vi "Dashboard Main.vi"() -> ()   [LabVIEW 2015]
uses:
  <vilib>/Utility/miscctls.llb/LVRowAndColumnTypeDef.ctl
  <vilib>/event_ctls.llb/eventvkey.ctl
  <vilib>/Rock Robotics/WPI/Dashboard/WPI_DashboardLogging Global.vi
  <vilib>/Rock Robotics/Network Tables/NT Read Numeric Array.vi
  <vilib>/Utility/config.llb/Write Key (String).vi
  <vilib>/Utility/config.llb/Write Key (I32).vi
  <vilib>/Utility/config.llb/NI_LVConfig.lvlib
panel:
  in  "TCP":refnum<k5>
  in  "Rec Mode":enum32{"Stop", "Record", "Playback"}(radio)
  in  "Vision":u16(ring) items=["Camera Off", "USB Camera SW", "USB Camera HW", "IP Camera"]
  out "Camera IP":string
  out "Image Message":string="Timeout in Camera Communications"
  in  "Dashboard Tab":T1(tab)
  in  "Select Auto":string(combo)
  out "NT Connection":bool
  in  "Camera Settings":T2={"Frame Rate"=30, "Compression"=30, "Size"=1} {"Frame Rate" scale=1.0..30.0; "Size" items=["640x480", "320x240", "160x120"]}
  out "MotorChart R":cluster{"Numeric":dbl, "Numeric":dbl}(graph)
  out "MotorChart L":T3(graph)
  out "MotorSliders R":cluster{"MotorSlide1":dbl, "MotorSlide2":dbl} {"MotorSlide2" scale=-1.0..1.0 scale format="%#_2e"; "MotorSlide1" scale=-1.0..1.0 scale format="%#_2e"}
  out "MotorSliders L":T4 {"MotorSlide4 2" scale=0.0..14.0 scale format="%#_2e"; "MotorSlide2" scale=-1.0..1.0 scale format="%#_2e"; "MotorSlide1" scale=-1.0..1.0 scale format="%#_2e"}
  out "Gyro":dbl(knob) scale=0.0..360.0
  out "JS1 Z":dbl(slide) scale=-1.0..1.0 scale format="%#_2e"
  out "JS1 Graph":cluster{"X":dbl, "Y":dbl}[](graph)
  out "JS1 Buttons":T5
  out "JS2 Z":dbl(slide) scale=-1.0..1.0 scale format="%#_2e"
  out "JS2 Graph":cluster{"X":dbl, "Y":dbl}[](graph)
  out "JS2 Buttons":T5
  out "Mode":T6(ring)=enum."Auto Disabled"
  in  "DB Camera Config":bool
  out "fps":dbl format="%#.1g"
  out "Mbps":dbl format="%#.1g"
  out "Mbps LED":bool
  in  "DB/String 9":string
  in  "DB/String 8":string
  in  "DB/String 7":string
  in  "DB/String 6":string
  in  "DB/String 5":string
  in  "DB/String 4":string
  in  "DB/String 3":string
  in  "DB/String 2":string
  in  "DB/String 1":string
  in  "DB/String 0":string
  in  "DB/Slider 0":dbl(slide) scale=0.0..5.0
  in  "DB/Slider 1":dbl(slide) scale=0.0..5.0
  in  "DB/Slider 2":dbl(slide) scale=0.0..5.0
  in  "DB/Slider 3":dbl(slide) scale=0.0..5.0
  out "DB/LED 3":bool
  out "DB/LED 2":bool
  out "DB/LED 1":bool
  out "DB/LED 0":bool
  in  "DB/Button 3":bool
  in  "DB/Button 2":bool
  in  "DB/Button 1":bool
  in  "DB/Button 0":bool caption="New Name"
  in  "Position_y":dbl
  in  "Position_x":dbl
  out "XY Graph":cluster{"X":dbl[], "Y":dbl[]}[](graph)
  in  "Reset_Camera":bool=TRUE
  in  "Enable_Camera":bool=TRUE
  in  "Test Slider":dbl(slide) scale=0.0..100.0 scale format="%#_3g"
  in  "On/Off":bool caption="Solenoid"
  in  "Test Name":u16(ring) items=["Select the test to run..."]
  in  "Test Tree":string(tree)
  in  "Motor":cluster{"Value":dbl, "Enable":bool} {"Value" scale=-1.0..1.0 scale format="%#_3g"}
  out "Progress":T7 {"Test Progress" scale=0.0..100.0}
  in  "Rev/Fwd":cluster{"Forward":bool, "Reverse":bool}
  in  "Test Ring":u16(ring) items=["Monochrome", "Color"]
  out "Cmd Status":string
  in  "Execute Command":bool
  in  "Command Params":string[][](table)
  in  "Command Selection":i32(listbox)
  in  "CheckList":i32(listbox)
  out "Tree":string(tree)
  out "Camera Image":T8(plugin-control)
  out "Background":bool
  # "Left"
  # "Front"
  # "Right"
  # "Battery"
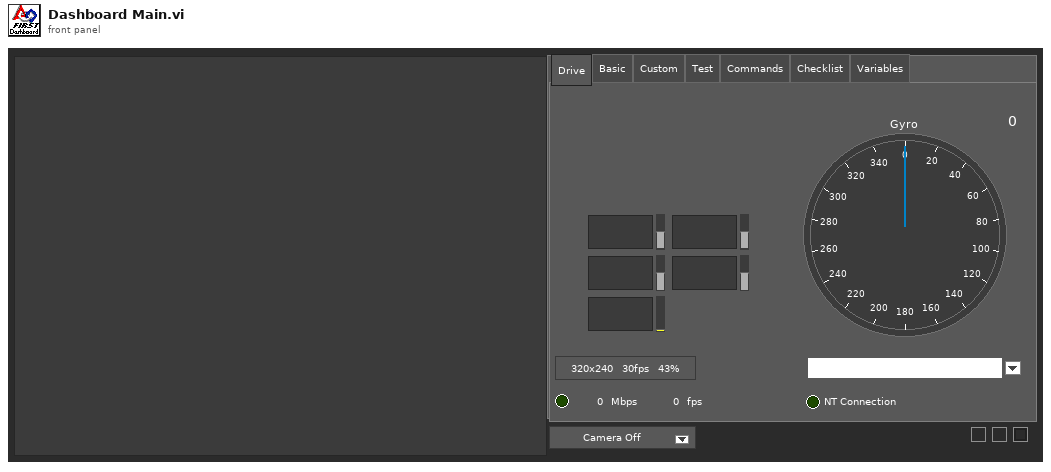
[diagram p1: front panel]
types:
  T1 = enum32{"Drive", "Basic", "Custom", "Test", "Commands", "Checklist", "Variables"}
  T2 = cluster{"Frame Rate":i32, "Compression":i32, "Size":u16}
  T3 = cluster{"Numeric":dbl, "Numeric":dbl, "Battery V":dbl}
  T4 = cluster{"MotorSlide1":dbl, "MotorSlide2":dbl, "MotorSlide4 2":dbl}
  T5 = cluster{bool, bool, bool, bool, bool, bool, bool, bool, bool, bool, bool, bool}
  T6 = enum8{"Tele-Op Disabled", "Tele-Op Enabled", "Auto Disabled", "Auto Enabled", "Test Disabled", "Test Enabled", "Disconnected", "No Code", "E-Stop"}
  T7 = cluster{"Test Progress":u8, "Test Progress Text":string}
  T8 = typedef "IMAQ Image.ctl" = refnum<image>
  T9 = cluster{"IDs":cluster{"RPC field ID":u16, "Unique ID":u16}, "String":string}
  T10 = enum32{"Drive", "Basic", "Custom", "Test", "Checklist", "Variables"}
  T11 = typedef "Image Type" = u32
  T12 = cluster{"Camera Image":refnum<vi>, "Dashboard Tab":refnum<vi>, "Background":refnum<vi>, "Vision":refnum<vi>, "Rec Mode":refnum<vi>, "Test Slider":refnum<vi>, "On/Off ":refnum<vi>, "Test Ring":refnum<vi>, "Rev/Fwd":refnum<vi>, "Test Name":refnum<vi>, "Motor":refnum<vi>, "Progress":refnum<vi>, "CheckList":refnum<vi>, "Tree":refnum<vi>, "Test Tree":refnum<vi>, "Command Params":refnum<vi>, "Command Selection":refnum<vi>, "Execute Command":refnum<vi>, "Cmd Status":refnum<vi>}
  T13 = cluster{"Error Strings":string, "Disable Counts":cluster{u16, u16}, "Rail Faults":cluster{u16, u16, u16}, "Robot IP":string, "DB Mode":u8, "Event Info":cluster{"Name":string, "Type":u8, "Number":u16, "Replay":u8}, "Camera Addr":string}
  T14 = cluster{"Storage":cluster{"Disk Free":u64, "RAM Block":u32, "RAM free":u32}, "CPU Utilization":cluster{"CPU % ISR":sgl, "CPU % Time Crit":sgl, "CPU % Timed Str":sgl, "CPU % High":sgl, "CPU % Above":sgl, "CPU % Normal":sgl, "CPU % Low":sgl}, "CAN":cluster{"% Bus Utilization":sgl, "Bus Off Cnt":u32, "TX_FIFO Full Cnt":u32, "Receive Error Cnt":u8, "Transmit Error Cnt":u8}, "HID":cluster{"HID Outputs":u32, "Rumble Low":u16, "Rumble High":u16}[]}
  T15 = cluster{"Status bits":cluster{"Test Mode":bool, "Autonomous":bool, "Enabled":bool, "Code Start":bool, "Brownout":bool, "Reserved 2":bool, "Reserved 3":bool, "E-Stop":bool}, "Code Trace":cluster{"Disabled":bool, "TeleOp":bool, "Auto":bool, "Test":bool}, "Controller Type":enum16{"unknown", "cRIO", "roboRio"}, "Code?":enum16{"unknown", "noCode", "code"}, "Battery V":dbl}
  T16 = cluster{"Control Bits":cluster{"TestMode":bool, "Autonomous":bool, "Enabled":bool, "FMS Present":bool, bool, bool, bool, "E-Stop":bool}, "Team Station ":u8, "Countdown":sgl, "Joystick Values":cluster{"Axes":dbl[], "Buttons":bool[], "POVs":i16[]}[]}
  T17 = cluster{"Axes":dbl[], "Buttons":bool[], "POVs":i16[]}[]
  T18 = cluster{"Axes":dbl[], "Buttons":bool[], "POVs":i16[]}
  T19 = cluster{"Buttons[0]":bool, "Buttons[1]":bool, "Buttons[2]":bool, "Buttons[3]":bool, "Buttons[4]":bool, "Buttons[5]":bool, "Buttons[6]":bool, "Buttons[7]":bool, "Buttons[8]":bool, "Buttons[9]":bool, "Buttons[10]":bool, "Buttons[11]":bool}
  T20 = typedef "NI_LVConfig.lvlib/Config Data RefNum.ctl" = refnum<k1>
  T21 = cluster{"Operation":enum16{"Update", "Clear"}, "Color Box":u32}[]
  T22 = typedef "eventvkey.ctl" = enum16{"ASCII", "Enter", "Return", "Shift", "Ctrl", "Alt", "Cmd", "Opt", "Caps", "NumLock", "Clear", "Break", "Up", "Down", "Left", "Right", "Insert", "Delete", "Home", "End", "PageUp", "PageDown", "Escape", "Help", "Pause", "ScrollLock", "F1", "F2", "F3", "F4", "F5", "F6", "F7", "F8", "F9", "F10", "F11", "F12", "F13", "F14", "F15", "F16", "F17", "F18", "F19", "F20", "F21", "F22", "F23", "F24", "Play", "VolumeUp", "VolumeDown", "Mute", "Two Byte Char"}
  T23 = cluster{"Image Size":bool, "Image Type":bool, "Pixel Value":bool, "ROI Information":bool, "Zoom Factor":bool}
  T24 = enum8{"Enabled", "Disabled", "Disabled and Grayed Out"}
  T25 = cluster{"Operation":enum16{"Update", "Clear"}, "Color Box":u32}
  T26 = typedef "LVRowAndColumnTypeDef.ctl" = cluster{"Row":i32, "Column":i32}
  T27 = cluster{"Shift":bool, "Ctrl":bool, "Alt":bool, "Cmd":bool, "Opt":bool}
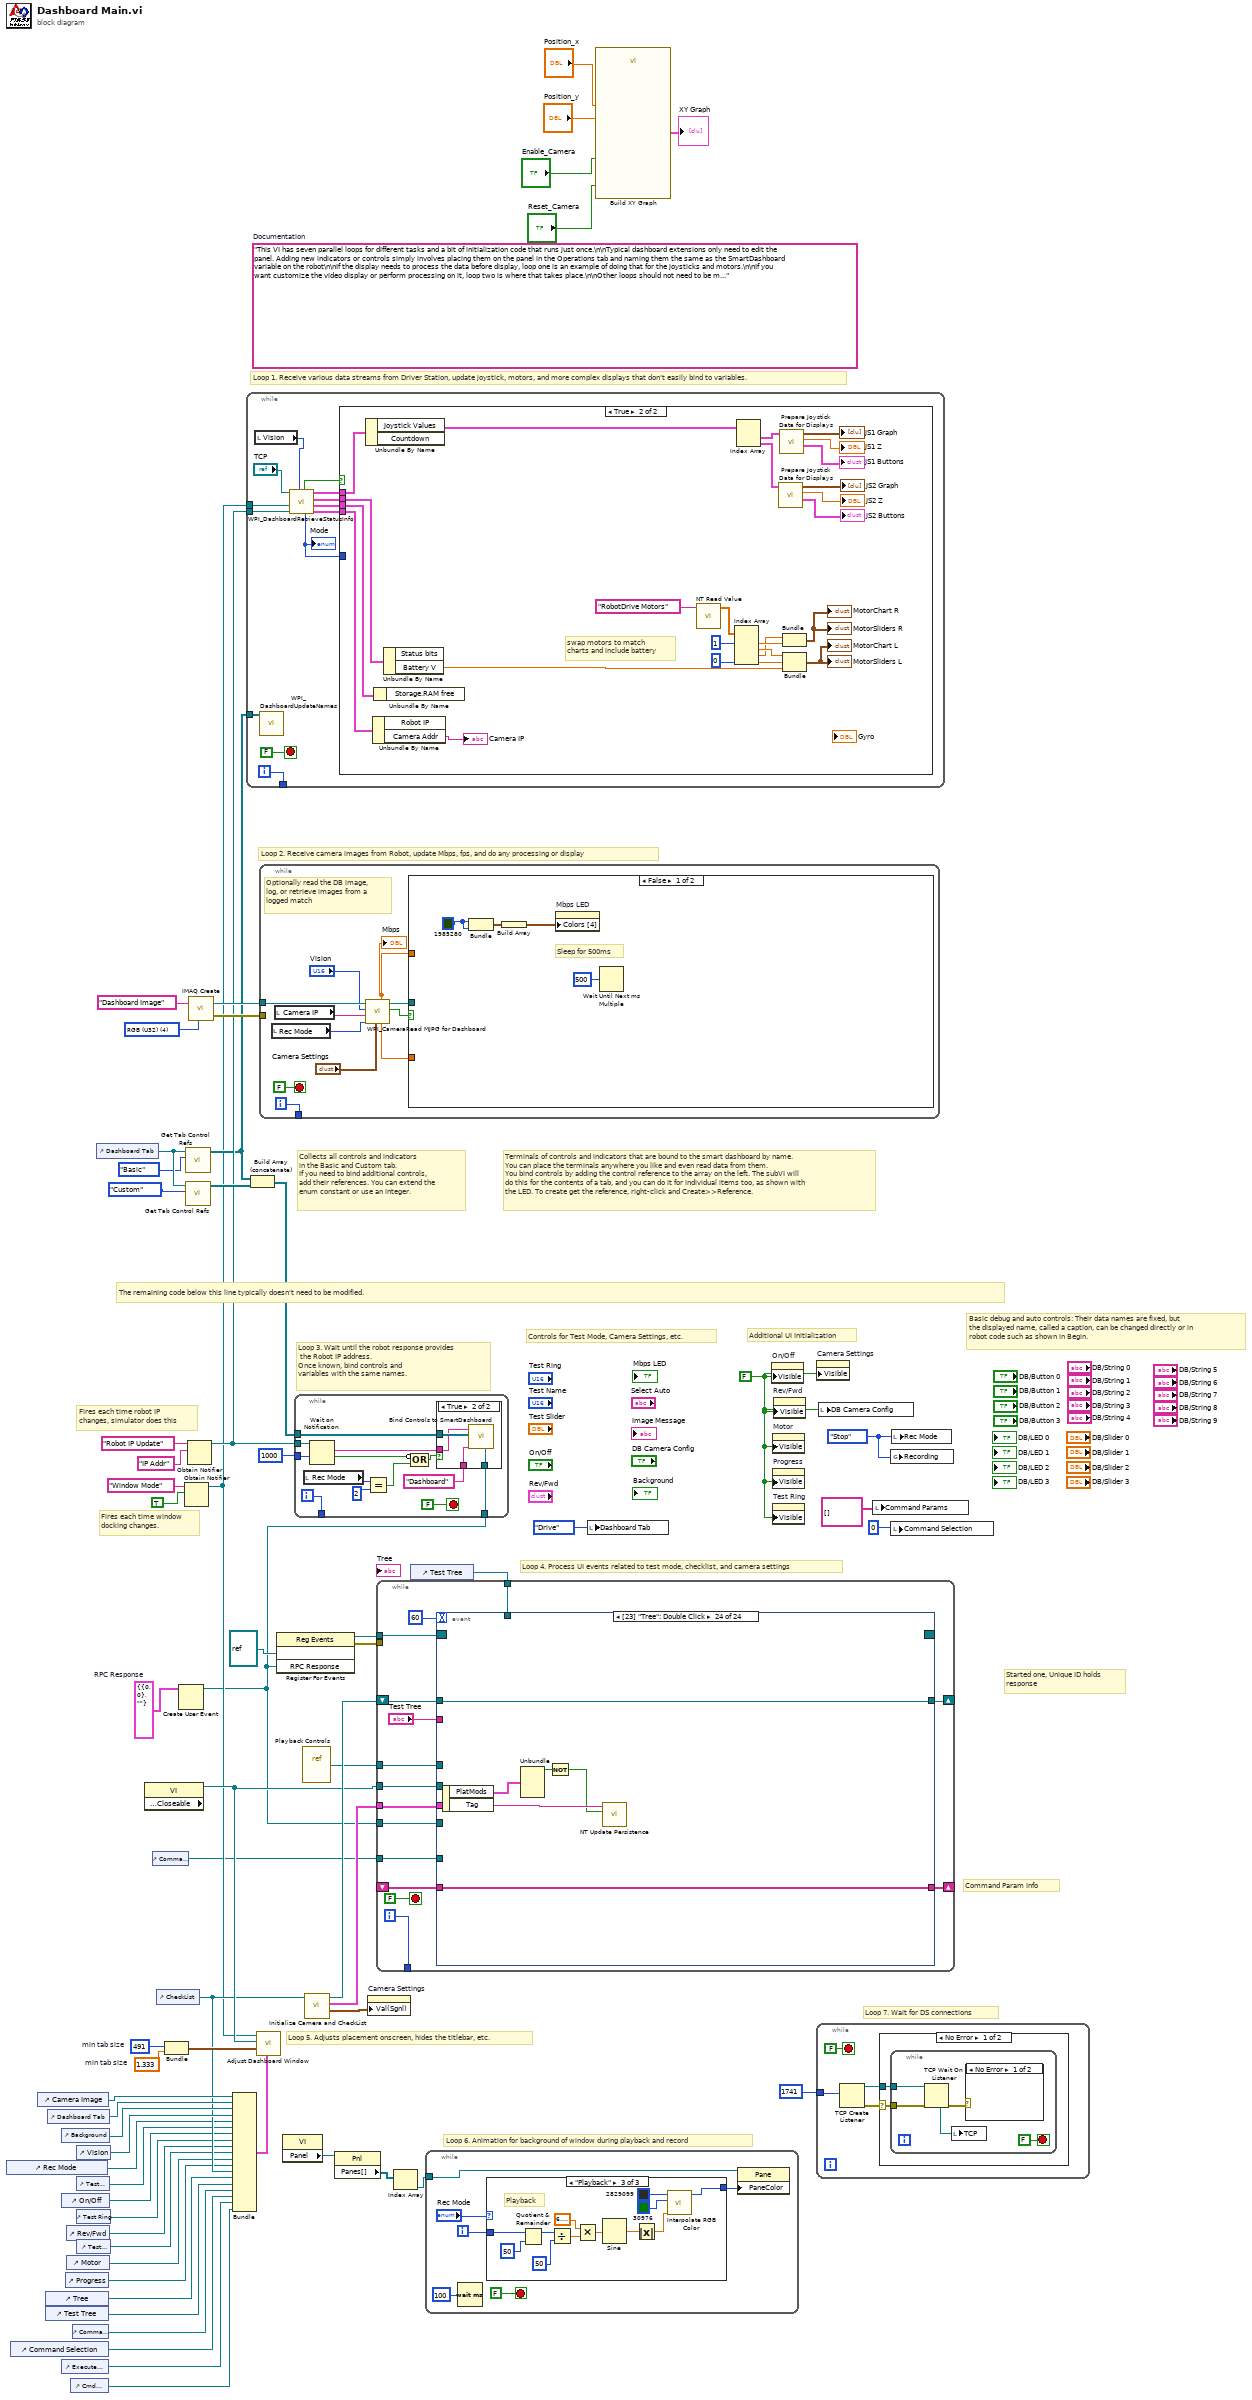
[diagram p0: block diagram]
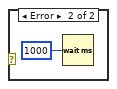
[diagram p2: hidden frame]
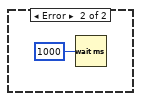
[diagram p3: hidden frame]
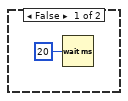
[diagram p4: hidden frame]
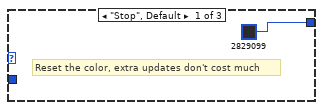
[diagram p5: hidden frame]
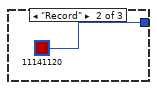
[diagram p6: hidden frame]
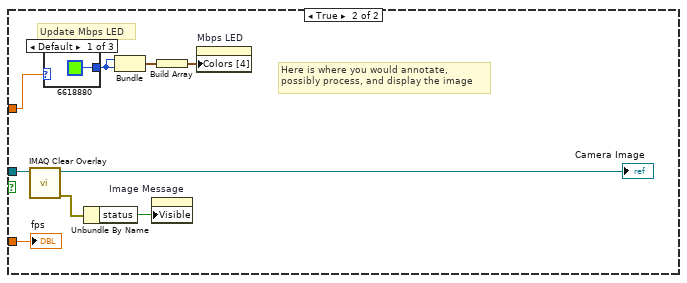
[diagram p8: hidden frame]
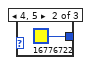
[diagram p9: hidden frame]
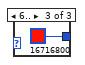
[diagram p10: hidden frame]
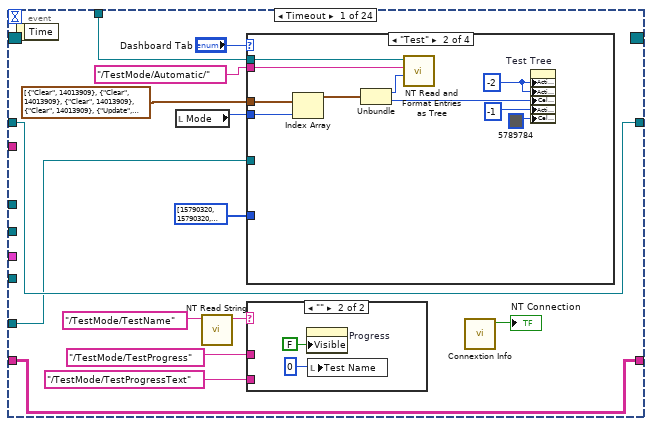
[diagram p11: hidden frame]
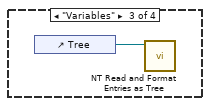
[diagram p13: hidden frame]
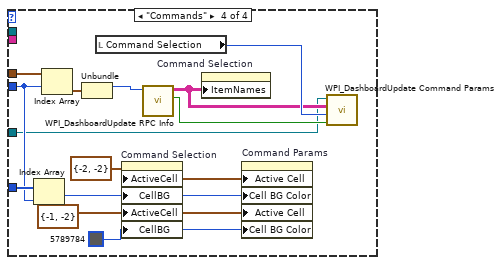
[diagram p14: hidden frame]
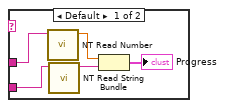
[diagram p15: hidden frame]
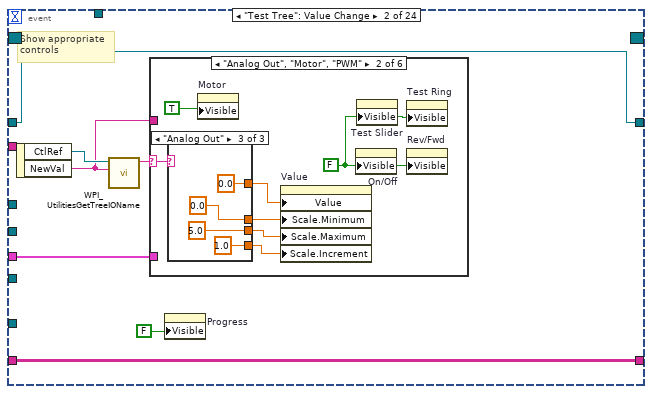
[diagram p16: hidden frame]
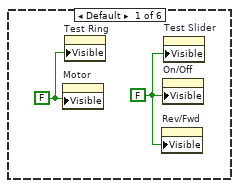
[diagram p17: hidden frame]
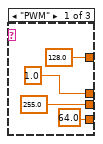
[diagram p18: hidden frame]
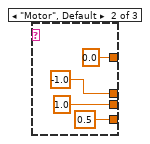
[diagram p19: hidden frame]
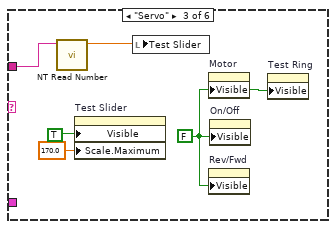
[diagram p20: hidden frame]
diagram:
  w12 = T9 {"IDs"={"RPC field ID"=0, "Unique ID"=0}, "String"=""}  # RPC Response
  w38 = 491  # min tab size
  w37 = 1.333  # min tab size
  w46 = enum32{"Stop", "Record", "Playback"}."Stop" ("Rec Mode")
  w20 = FALSE ("Visible")
  (unwired) "This VI has seven parallel loops for different tasks and a bit of initialization code that runs just once.\n\nTypical dashboard extensions only need to edit the panel. Adding new indicators or controls simply involves placing them on the panel in the Operations tab and naming them the same as the SmartDashboard variable on the robot\n\nIf the display needs to process the data before display, loop one is an example of doing that for the joysticks and motors.\n\nIf you want customize the video display or perform processing on it, loop two is where that takes place.\n\nOther loops should not need to be modified. They are pretty standard, and document the task they perform."  # Documentation
  w66 = T11 4 items=["Grayscale (U8)", "Grayscale (I16)", "Grayscale (SGL)", "Complex (CSG)", "RGB (U32)", "HSL (U32)", "RGB (U64)"] ("Image Type")
  # "Command Param Info"
  # "Started one, Unique ID holds\nresponse"
  # "Loop 7. Wait for DS connections"
  # "Basic debug and auto controls: Their data names are fixed, but\nthe displayed name, called a caption, can be changed directly or in\nrobot code such as shown in Begin."
  # "Controls for Test Mode, Camera Settings, etc."
  # "Additional UI Initialization"
  # "Loop 6. Animation for background of window during playback and record"
  # "Fires each time robot IP\nchanges, simulator does this"
  # "Fires each time window\ndocking changes."
  # "Collects all controls and indicators\nin the Basic and Custom tab.\nIf you need to bind additional controls,\nadd their references. You can extend the\nenum constant or use an integer."
  # "The remaining code below this line typically doesn't need to be modified."
  # "Loop 4. Process UI events related to test mode, checklist, and camera settings"
  # "Terminals of controls and indicators that are bound to the smart dashboard by name.\nYou can place the terminals anywhere you like and even read data from them.\nYou bind controls by adding the control reference to the array on the left. The subVI will\ndo this for the contents of a tab, and you can do it for individual items too, as shown with\nthe LED. To create get the reference, right-click and Create>>Reference."
  # "Loop 3. Wait until the robot response provides\n the Robot IP address.\nOnce known, bind controls and\nvariables with the same names."
  # "Loop 5. Adjusts placement onscreen, hides the titlebar, etc."
  # "Loop 1. Receive various data streams from Driver Station, update joystick, motors, and more complex displays that don't easily bind to variables."
  # "Loop 2. Receive camera images from Robot, update Mbps, fps, and do any processing or display"
  n1 = control-ref of="Rec Mode"() -> (w26:refnum<vi>)
  n2 = control-ref of="Command Selection"() -> (w11:refnum<vi>)
  n3 = control-ref of="Camera Image"() -> (w41:refnum<vi>)
  n4 = control-ref of="Tree"() -> (w30:refnum<vi>)
  n5 = control-ref of="Test Tree"() -> (w29:refnum<vi>)
  n6 = control-ref of="Dashboard Tab"() -> (w40:refnum<vi>)
  n7 = control-ref of="Execute Command"() -> (w13:refnum<vi>)
  n8 = control-ref of="Background"() -> (w35:refnum<vi>)
  n9 = control-ref of="On/Off"() -> (w24:refnum<vi>)
  n10 = control-ref of="Progress"() -> (w21:refnum<vi>)
  n11 = control-ref of="Rev/Fwd"() -> (w22:refnum<vi>)
  n12 = control-ref of="Motor"() -> (w27:refnum<vi>)
  n13 = control-ref of="Cmd Status"() -> (w7:refnum<vi>)
  n14 = control-ref of="Command Params"() -> (w14:refnum<vi>)
  n15 = control-ref of="Test Slider"() -> (w25:refnum<vi>)
  n16 = control-ref of="Vision"() -> (w39:refnum<vi>)
  n17 = control-ref of="Test Ring"() -> (w23:refnum<vi>)
  n18 = control-ref of="Test Name"() -> (w28:refnum<vi>)
  n19 = control-ref of="Dashboard Tab"() -> (w44:refnum<vi>)
  n20 = property class="VI" props=["Front Panel.Closeable"]() -> (reference out=w45:refnum<vi>)  [unwired: 2 in, 2 out]
  n21 = control-ref of="Command Params"() -> (w6:refnum<vi>)
  n22 = control-ref of="CheckList"() -> (w31:refnum<vi>)
  n23 = Bundle("min tab size"=w38, "min tab size"=w37) -> (w36:cluster{"min tab size":i32, "min tab size":dbl})  [unwired: 1 in]
  n24 = Create User Event(user event datatype=w12) -> (user event=w8:refnum<user-event>)  [unwired: 1 in, 1 out]
  n25 = Obtain Notifier(name (unnamed)="Window Mode", notification data type=TRUE) -> (notifier out=w17:refnum<notifier>)  [unwired: 2 in, 2 out]
  n26 = call <vilib>:"Get Tab Control Refs.vi"("Page Index"=T10."Basic" ("Dashboard Tab"), "TabControl in"=w44) -> ("ControlsOnPage"=w18:refnum<vi>[])  [unwired: 9 in]
  n27 = call <vilib>:"Get Tab Control Refs.vi"("Page Index"=T10."Custom" ("Dashboard Tab"), "TabControl in"=w44) -> ("ControlsOnPage"=w43:refnum<vi>[])  [unwired: 9 in]
  n28 = Obtain Notifier(name (unnamed)="Robot IP Update", notification data type="IP Addr" ("name (unnamed)")) -> (notifier out=w19:refnum<notifier>)  [unwired: 2 in, 2 out]
  n29 = call "IMAQ Create"("Image Name"="Dashboard Image", "Image Type"=w66) -> ("New Image"=w64:T8, "error out"=w63:errorcluster)  [unwired: 2 in, 1 out]
  n30 = Bundle("Camera Image"=w41, "Dashboard Tab"=w40, "Background"=w35, "Vision"=w39, "Rec Mode"=w26, "Test Slider"=w25, "On/Off"=w24, "Test Ring"=w23, "Rev/Fwd"=w22, "Test Name"=w28, "Motor"=w27, "Progress"=w21, "CheckList"=w31, "Tree"=w30, "Test Tree"=w29, "Command Params"=w14, "Command Selection"=w11, "Execute Command"=w13, "Cmd Status"=w7) -> (w32:T12)  [unwired: 1 in]
  n31 = while {
    tunnel: [w78] -> _
    tunnel: w19 -> [w72]
    tunnel: w18 -> [w71]
    tunnel: w17 -> [w67]
    i -> [w78]
    stop <- FALSE stop-if-true
    n32 = local read "Vision"() -> (w69:u16)
    n33 = call <vilib>:"WPI_DashboardUpdateNames.vi"("Controls on Tab"=w71) -> ()  [unwired: 11 in]
    n34 = call <vilib>:"WPI_DashboardRetrieveStatusInfo.vi"("Vision"=w69, "Binding Refnum"=w72, "Window Mode Notifier"=w67, "TCP Cnx"="TCP") -> ("Power and Errors"=w73:T13, "Robot Metrics"=w76:T14, "Status Info"=w77:T15, "Control Info"=w74:T16, "Robot Mode"=w70:T6, "Process?"=w75:bool)  [unwired: 2 in]
    "Mode" <- w70
    n35 = case shown="True" w75 {
      tunnel: w77 -> [_ w105]
      tunnel: w76 -> [_ w104]
      tunnel: w74 -> [_ w103]
      tunnel: w73 -> [_ w102]
      tunnel: w70 -> [_ _]
      frame False {
        n36 = Wait (ms)(milliseconds to wait=u32 20) -> ()  [unwired: 1 out]
      }
      frame True {
        # "swap motors to match\ncharts and include battery"
        n37 = Unbundle By Name(w103) -> ("Joystick Values"=w92:T17)  [unwired: 1 out]
        n38 = Unbundle By Name(w102) -> ("Camera Addr"=→"Camera IP":string)  [unwired: 1 out]
        n39 = Unbundle By Name(w104) -> ()  [unwired: 1 out]
        n40 = Unbundle By Name(w105) -> ("Battery V"=w93:dbl)  [unwired: 1 out]
        n41 = call-poly <vilib>:"NT Read Value.vi"("Name"="RobotDrive Motors") -> ("Numeric Array"=w81:dbl[])  [unwired: 9 in, 1 out]
        n42 = Index Array(array=w81, index #1=1, index #4=0) -> (element #1=w97:dbl, element #2=w98:dbl, element #3=w96:dbl, element #4=w101:dbl)  [unwired: 2 in]
        n43 = Index Array(array=w92) -> (element #1=w91:T18, element #2=w86:T18)  [unwired: 2 in]
        n44 = call "Prepare Joystick Data for Displays.vi"("Joystick Values"=w86) -> ("Buttons"=→"JS2 Buttons":T19, "Z Axis"=→"JS2 Z":dbl, "Cartesian Data"=→"JS2 Graph":cluster{"X axis":dbl, "X axis":dbl}[])  [unwired: 8 in]
        n45 = call "Prepare Joystick Data for Displays.vi"("Joystick Values"=w91) -> ("Buttons"=→"JS1 Buttons":T19, "Z Axis"=→"JS1 Z":dbl, "Cartesian Data"=→"JS1 Graph":cluster{"X axis":dbl, "X axis":dbl}[])  [unwired: 8 in]
        n46 = Bundle("Numeric"=w96, "Numeric"=w97) -> (→"MotorChart R" →"MotorSliders R":cluster{"Numeric":dbl, "Numeric":dbl})  [unwired: 1 in]
        n47 = Bundle("Numeric"=w98, "Numeric"=w101, "Battery V"=w93) -> (→"MotorChart L" →"MotorSliders L":T3)  [unwired: 1 in]
      }
    }
  }
  n48 = Build Array (concatenate)(w18, w43) -> (w42:refnum<vi>[])
  n49 = call "Adjust Dashboard Window.vi"("Sizing Refnums"=w32, "Size Constraints"=w36, "VI"=w45, "WIn Mode"=w17) -> ()  [unwired: 8 in]
  n50 = while {
    tunnel: w64 -> [w114]
    tunnel: w63 -> [_]
    tunnel: [w115] -> _
    i -> [w115]
    stop <- FALSE stop-if-true
    # "Optionally read the DB image,\nlog, or retrieve images from a\nlogged match"
    n51 = local read "Rec Mode"() -> (w109:enum32{"Stop", "Record", "Playback"})
    n52 = local read "Camera IP"() -> (w107:string)
    n53 = call <vilib>:"WPI_CameraRead MJPG for Dashboard.vi"("Camera Settings"="Camera Settings", "Rec Mode"=w109, "Camera IP"=w107, "Camera Mode"="Vision", "Refnum in"=w114) -> ("Active"=w112:bool, "Refnum out"=w113:T8, "FPS"=w111:dbl, "Bandwidth (Mbps)"=w106:dbl)  [unwired: 3 in]
    "Mbps" <- w106
    n54 = case shown="False" w112 {
      tunnel: w113 -> [_ w124]
      tunnel: w106 -> [_ w123]
      tunnel: w111 -> [_ w121]
      frame False {
        w117 = u32 1985280 ("Color Box")
        # "Sleep for 500ms"
        n55 = Bundle("Color Box"=w117, "Color Box"=w117) -> (w119:cluster{"Color Box":u32, "Color Box":u32})  [unwired: 1 out]
        n56 = Build Array(w119) -> (w118:cluster{"Color Box":u32, "Color Box":u32}[])
        n57 = property on="Mbps LED" class="Bool (strict)"("Colors [4]"=w118) -> ()  [unwired: 2 in, 2 out]
        n58 = Wait Until Next ms Multiple(millisecond multiple=u32 500) -> ()  [unwired: 1 out]
      }
      frame True {
        # "Here is where you would annotate,\npossibly process, and display the image"
        # "Update Mbps LED"
        n59 = call "IMAQ Clear Overlay"("Image"=w124) -> ("error out"=w128:errorcluster, "Image Out"=→"Camera Image":T8)  [unwired: 2 in, 7 out]
        n60 = case shown="Default" w123 {
          tunnel: [u32 6618880 ("Color Box") u32 16776722 ("Color Box") u32 16716800 ("Color Box")] -> w125
          frame Default {
          }
          frame 4, 5 {
          }
          frame 6.. {
          }
        }
        n61 = Unbundle By Name(w128) -> ("status"=w129:bool)
        n62 = Bundle("Color Box"=w125, "Color Box"=w125) -> (w127:cluster{"Color Box":u32, "Color Box":u32})  [unwired: 1 out]
        n63 = property on="Image Message" class="Str"("Visible"=w129) -> ()  [unwired: 2 in, 2 out]
        n64 = Build Array(w127) -> (w126:cluster{"Color Box":u32, "Color Box":u32}[])
        n65 = property on="Mbps LED" class="Bool (strict)"("Colors [4]"=w126) -> ()  [unwired: 2 in, 2 out]
        "fps" <- w121
      }
    }
  }
  n66 = register-events(refnum<vi> refnum, w8) -> (reference out=w50:refnum<event-registration>, error out=w49:errorcluster)  [unwired: 2 in]
  n67 = property class="VI"() -> ("Panel"=w53:refnum<vi>)  [unwired: 2 in, 2 out]
  n68 = while {
    tunnel: w42 -> [w145]
    tunnel: w19 -> [w143]
    tunnel: [w141] -> _
    tunnel: u32 1000 ("milliseconds to wait") -> [w140]
    tunnel: w8 -> [w133]
    i -> [w141]
    stop <- FALSE stop-if-true
    n69 = local read "Rec Mode"() -> (w136:enum32{"Stop", "Record", "Playback"})
    n70 = Wait on Notification(notifier=w143, timeout in ms (-1)=w140) -> (notification=w142:string, timed out?=w138:bool)  [unwired: 2 in, 2 out]
    n71 = Equal?(x=w136, y=u16 2 ("Rec Mode")) -> (x = y?=w137:bool)
    n72 = Compound Arithmetic op=OR(invert w138, w137) -> (w139:bool)
    n73 = case shown="True" w139 {
      tunnel: w145 -> [_ w149]
      tunnel: w142 -> [_ w148]
      tunnel: "Dashboard" -> [_ w147]
      tunnel: w133 -> [_ w146]
      frame False {
      }
      frame True {
        n74 = call <vilib>:"Bind Controls to SmartDashboard.vi"("RPC ref"=w146, "Client Name"=w147, "Bound Control Refs"=w149, "Server IP Address"=w148) -> ()  [unwired: 8 in]
      }
    }
  }
  n75 = vi-ref "Playback Controls.vi"() -> (w51:refnum<vi>)
  n76 = call "Initialize Camera and CheckList.vi"("ListBox in"=w31) -> ("Cluster"=w57:cluster{"value":i32, "value":i32, "index":i32}, "Array"=w58:cluster{string[]}[], "File Refnum"=w56:T20)  [unwired: 8 in]
  n77 = property class="Pnl"(reference=w53) -> ("Panes[]"=w54:refnum<vi>[])  [unwired: 1 in, 2 out]
  n78 = property on="Camera Settings" class="Clust (strict)"("Val(Sgnl)"=w57) -> ()  [unwired: 2 in, 2 out]
  n79 = Index Array(array=w54) -> (element=w52:refnum<vi>)  [unwired: 1 in]
  n80 = control-ref of="Test Tree"() -> (w55:refnum<vi>)
  n81 = while {
    tunnel: w58 -> [w161]
    shift-right: [w160] -> _
    shift-left: w56 -> [w159]
    tunnel: [w158] -> _
    tunnel: w55 -> [w157]
    tunnel: w51 -> [w156]
    tunnel: w50 -> [w155]
    tunnel: w49 -> [_]
    tunnel: w45 -> [w154]
    tunnel: w8 -> [w153]
    tunnel: w6 -> [w152]
    shift-right: [w151] -> _
    shift-left: _ -> [w150]
    i -> [w158]
    stop <- FALSE stop-if-true
    n82 = event shown="[23] \"Tree\": Double Click" {
      selector: w155 -> [_ _ _ _ _ _ _ _ _ _ _ _ _ _ _ _ _ _ _ _ _ _ _ _]
      dyn-events: [_ _ _ _ _ _ _ _ _ _ _ _ _ _ _ _ _ _ w470 _ _ _ _ _] -> _
      timeout: u32 60 ("milliseconds to wait") -> [_ _ _ _ _ _ _ _ _ _ _ _ _ _ _ _ _ _ _ _ _ _ _ _]
      tunnel: w157 -> [w174 _ _ _ _ _ _ _ _ _ _ _ _ _ _ _ _ _ _ _ _ _ _ _]
      tunnel: "Test Tree" -> [_ _ _ _ _ _ _ _ _ _ _ _ _ w433 w442 w445 w450 w459 _ _ _ _ _ _]
      tunnel: w161 -> [_ w212 _ _ _ _ _ _ _ _ _ w395 w426 _ _ _ _ _ _ _ _ _ _ _]
      tunnel: [w171 w211 w315 w321 w331 w335 w341 w353 w361 w367 w380 w394 w419 w432 w440 w444 w449 w458 w472 w488 w490 w498 w509 w514] -> w160
      tunnel: w159 -> [w171 w211 w315 w321 w331 w335 w341 w353 w361 w367 w380 w393 w419 w432 w440 w444 w449 w458 w472 w488 w490 w498 w509 w514]
      tunnel: w156 -> [_ _ _ _ _ _ _ _ _ _ _ _ _ _ _ _ _ _ w473 _ w493 _ _ _]
      tunnel: w154 -> [_ _ _ _ _ _ _ _ _ _ _ _ _ _ _ _ _ _ w468 _ _ _ _ _]
      tunnel: w153 -> [_ _ _ _ _ _ _ _ _ _ _ _ _ _ _ _ _ _ w464 _ _ _ _ _]
      tunnel: w152 -> [w166 _ _ _ _ _ w339 _ _ _ _ _ _ _ _ _ _ _ _ _ _ _ _ _]
      tunnel: [w165 w210 w314 w320 w330 w336 w337 w347 w358 w366 w379 w392 w418 w431 w439 w443 w448 w457 w463 w486 w489 w494 w502 w515] -> w151
      tunnel: w150 -> [w165 w210 w314 w320 w330 w336 w337 _ _ w366 w379 w392 w418 w431 w439 w443 w448 w457 w463 w486 w489 w494 w502 w515]
      event Timeout {
        n83 = event-data() -> ()  [unwired: 1 in, 1 out]
        n84 = local read "Mode"() -> (w168:T6)
        n85 = call <vilib>:"NT Read String.vi"("Name"="/TestMode/TestName") -> ("String"=w177:string)  [unwired: 9 in, 1 out]
        n86 = case shown="\"Test\"" "Dashboard Tab" {
          tunnel: w174 -> [_ w188 _ _]
          tunnel: "/TestMode/Automatic/" ("Name Pattern") -> [_ w187 _ _]
          tunnel: T21 [{"Operation"=enum."Clear", "Color Box"=14013909}, {"Operation"=enum."Clear", "Color Box"=14013909}, {"Operation"=enum."Clear", "Color Box"=14013909}, {"Operation"=enum."Clear", "Color Box"=14013909}, {"Operation"=enum."Update", "Color Box"=14013909}, {"Operation"=enum."Update", "Color Box"=16777215}, {"Operation"=enum."Clear", "Color Box"=14013909}, {"Operation"=enum."Clear", "Color Box"=14013909}, {"Operation"=enum."Clear", "Color Box"=14013909}] -> [_ w180 _ w197]
          tunnel: w168 -> [_ w179 _ w196]
          tunnel: u32[] [15790320, 15790320, 15790320, 15790320, 16777215, 16777215, 15790320, 15790320, 15790320] -> [_ _ _ w202]
          tunnel: w166 -> [_ _ _ w190]
          frame "Custom", Default {
          }
          frame "Test" {
            w186 = -2 ("Active Item:Row Number")
            n87 = Index Array(array=w180, index=w179) -> (element=w181:T25)
            n88 = Unbundle(w181) -> ("Operation"=w182:enum16{"Update", "Clear"}, "Color Box"=w183:u32)
            n89 = call <vilib>:"NT Read and Format Entries as Tree.vi"("Operation"=w182, "Name Pattern"=w187, "Tree Refnum"=w188) -> ()  [unwired: 7 in, 2 out]
            n90 = property on="Test Tree" class="Tree (strict)"("Active Item Row Number"=w186, "ActiveColNum"=w186, "CellBG"=w183, "Active Item Row Number"=-1 ("Active Item:Row Number"), "CellBG"=u32 5789784 ("Color Box")) -> ()  [unwired: 2 in, 2 out]
          }
          frame "Variables" {
            n91 = control-ref of="Tree"() -> (w189:refnum<vi>)
            n92 = call <vilib>:"NT Read and Format Entries as Tree.vi"("Tree Refnum"=w189) -> ()  [unwired: 9 in, 2 out]
          }
          frame "Commands" {
            w198 = u32 5789784 ("Color Box")
            w199 = T26 {"Row"=-1, "Column"=-2} ("Active Cell:Active Cell")
            w201 = T26 {"Row"=-2, "Column"=-2} ("Active Cell:Active Cell")
            n93 = Index Array(array=w202, index=w196) -> (element=w200:u32)
            n94 = Index Array(array=w197, index=w196) -> (element=w195:T25)
            n95 = Unbundle(w195) -> ("Operation"=w194:enum16{"Update", "Clear"})  [unwired: 1 out]
            n96 = local read "Command Selection"() -> (w193:i32)
            n97 = property on="Command Selection" class="MCListbox (strict)"("ActiveCell"=w201, "CellBG"=w200, "ActiveCell"=w199, "CellBG"=w198) -> ()  [unwired: 2 in, 2 out]
            n98 = call <vilib>:"WPI_DashboardUpdate RPC Info.vi"("Operation"=w194) -> ("update"=w192:bool, "commands"=w191:string[][])  [unwired: 9 in]
            n99 = property on="Command Selection" class="MCListbox (strict)"("ItemNames"=w191) -> ()  [unwired: 2 in, 2 out]
            n100 = property on="Command Params" class="Tbl (strict)"("Active Cell"=w201, "Cell BG Color"=w200, "Active Cell"=w199, "Cell BG Color"=w198) -> ()  [unwired: 2 in, 2 out]
            n101 = call <vilib>:"WPI_DashboardUpdate Command Params.vi"("Update"=w192, "NewVal"=w193, "Commands"=w191, "Param Tbl"=w190) -> ()  [unwired: 7 in, 1 out]
          }
        }
        n102 = case shown="\"\"" w177 {
          tunnel: "/TestMode/TestProgress" ("Name") -> [w204 _]
          tunnel: "/TestMode/TestProgressText" ("Name") -> [w203 _]
          frame Default {
            n103 = call <vilib>:"NT Read Number.vi"("Name"=w204) -> ("Numeric"=w205:dbl)  [unwired: 9 in, 1 out]
            n104 = call <vilib>:"NT Read String.vi"("Name"=w203) -> ("String"=w206:string)  [unwired: 9 in, 1 out]
            n105 = Bundle("Numeric"=w205, "String"=w206) -> (→"Progress":cluster{"Numeric":dbl, "String":string})  [unwired: 1 in]
          }
          frame "" {
            n106 = property on="Progress" class="Clust (strict)"("Visible"=FALSE) -> ()  [unwired: 2 in, 2 out]
            n107 = local write "Test Name"(u16 0) -> ()
          }
        }
        n108 = call <vilib>:"Connextion Info.vi"() -> ("Connected"=→"NT Connection":bool)  [unwired: 10 in, 1 out]
      }
      event "Test Tree": Value Change {
        # "Show appropriate\ncontrols"
        n109 = event-data() -> ("CtlRef"=w215:refnum<vi>, "NewVal"=w213:string)  [unwired: 1 in]
        n110 = call <vilib>:"WPI_UtilitiesGetTreeIOName.vi"("NewVal"=w213, "TreeControl in"=w215) -> ("I/O Name"=w216:string)  [unwired: 9 in]
        n111 = case shown="\"Analog Out\", \"Motor\", \"PWM\"" w216 {
          selector: w216 -> [_ w223 _ w245 w254 _]
          tunnel: w213 -> [_ _ w242 w244 _ w261]
          tunnel: w212 -> [_ _ _ _ _ w260]
          frame Default {
            w218 = FALSE ("Visible")
            w217 = FALSE ("Visible")
            n112 = property on="Motor" class="Clust (strict)"("Visible"=w217) -> ()  [unwired: 2 in, 2 out]
            n113 = property on="Test Ring" class="Ring (strict)"("Visible"=w217) -> ()  [unwired: 2 in, 2 out]
            n114 = property on="Rev/Fwd" class="Clust (strict)"("Visible"=w218) -> ()  [unwired: 2 in, 2 out]
            n115 = property on="On/Off" class="Bool (strict)"("Visible"=w218) -> ()  [unwired: 2 in, 2 out]
            n116 = property on="Test Slider" class="Slide (strict)"("Visible"=w218) -> ()  [unwired: 2 in, 2 out]
          }
          frame "Analog Out", "Motor", "PWM" {
            w224 = FALSE ("Visible")
            n117 = case shown="\"Analog Out\"" w223 {
              tunnel: [1.0 ("Value") -1.0 ("Value") 0.0 ("Value")] -> w222
              tunnel: [255.0 ("Value") 1.0 ("Value") 5.0 ("Value")] -> w221
              tunnel: [128.0 ("Value") 0.0 ("Value") 0.0 ("Value")] -> w220
              tunnel: [64.0 ("Value") 0.5 ("Value") 1.0 ("Value")] -> w219
              frame "PWM" {
              }
              frame "Motor", Default {
              }
              frame "Analog Out" {
              }
            }
            n118 = property on="Motor" class="Clust (strict)"("Visible"=TRUE) -> ()  [unwired: 2 in, 2 out]
            n119 = property on="Value" class="Slide (strict)"("Value"=w220, "Scale.Minimum"=w222, "Scale.Maximum"=w221, "Scale.Increment"=w219) -> ()  [unwired: 2 in, 2 out]
            n120 = property on="On/Off" class="Bool (strict)"("Visible"=w224) -> ()  [unwired: 2 in, 2 out]
            n121 = property on="Test Slider" class="Slide (strict)"("Visible"=w224) -> ()  [unwired: 2 in, 2 out]
            n122 = property on="Test Ring" class="Ring (strict)"("Visible"=w224) -> ()  [unwired: 2 in, 2 out]
            n123 = property on="Rev/Fwd" class="Clust (strict)"("Visible"=w224) -> ()  [unwired: 2 in, 2 out]
          }
          frame "Servo" {
            w240 = FALSE ("Visible")
            n124 = call <vilib>:"NT Read Number.vi"("Name"=w242) -> ("Numeric"=w241:dbl)  [unwired: 9 in, 1 out]
            n125 = property on="Test Slider" class="Slide (strict)"("Visible"=TRUE, "Scale.Maximum"=170.0 ("Scale.Range:Maximum")) -> ()  [unwired: 2 in, 2 out]
            n126 = local write "Test Slider"(w241) -> ()
            n127 = property on="Motor" class="Clust (strict)"("Visible"=w240) -> ()  [unwired: 2 in, 2 out]
            n128 = property on="Rev/Fwd" class="Clust (strict)"("Visible"=w240) -> ()  [unwired: 2 in, 2 out]
            n129 = property on="On/Off" class="Bool (strict)"("Visible"=w240) -> ()  [unwired: 2 in, 2 out]
            n130 = property on="Test Ring" class="Ring (strict)"("Visible"=w240) -> ()  [unwired: 2 in, 2 out]
          }
          frame "Relay", "Solenoid" {
            w243 = FALSE ("Visible")
            n131 = property on="Motor" class="Clust (strict)"("Visible"=w243) -> ()  [unwired: 2 in, 2 out]
            n132 = property on="Test Slider" class="Slide (strict)"("Visible"=w243) -> ()  [unwired: 2 in, 2 out]
            n133 = Search and Replace String(input string=w244, search string="/Value  **", replace string="/Direction") -> (result string=w250:string)  [unwired: 5 in, 3 out]
            n134 = property on="Test Ring" class="Ring (strict)"("Visible"=w243) -> ()  [unwired: 2 in, 2 out]
            n135 = call <vilib>:"NT Read String.vi"("Name"=w250) -> ("String"=w248:string)  [unwired: 9 in, 1 out]
            n136 = Equal?(x="Both directions", y=w248) -> (x = y?=w246:bool)
            n137 = Not(x=w246) -> (.not. x?=w247:bool)
            n138 = property on="Rev/Fwd" class="Clust (strict)"("Visible"=w246) -> ()  [unwired: 2 in, 2 out]
            n139 = property on="On/Off" class="Bool (strict)"("Visible"=w247, "Caption.Text"=w245) -> ()  [unwired: 2 in, 2 out]
          }
          frame "Compressor", "Digital Out" {
            w253 = FALSE ("Visible")
            # "Get direction and finish"
            n140 = property on="Motor" class="Clust (strict)"("Visible"=w253) -> ()  [unwired: 2 in, 2 out]
            n141 = property on="Test Slider" class="Slide (strict)"("Visible"=w253) -> ()  [unwired: 2 in, 2 out]
            n142 = property on="Test Ring" class="Ring (strict)"("Visible"=w253) -> ()  [unwired: 2 in, 2 out]
            n143 = property on="On/Off" class="Bool (strict)"("Visible"=TRUE, "Caption.Text"=w254) -> ()  [unwired: 2 in, 2 out]
            n144 = property on="Rev/Fwd" class="Clust (strict)"("Visible"=FALSE) -> ()  [unwired: 2 in, 2 out]
          }
          frame "Camera" {
            n145 = call <vilib>:"Get Last Path Segment.vi"("String in"=w261) -> ("String out"=w262:string)  [unwired: 10 in]
            n146 = property on="On/Off" class="Bool (strict)"("Visible"=FALSE) -> ()  [unwired: 2 in, 2 out]
            n147 = property on="Motor" class="Clust (strict)"("Visible"=FALSE) -> ()  [unwired: 2 in, 2 out]
            n148 = property on="Rev/Fwd" class="Clust (strict)"("Visible"=FALSE) -> ()  [unwired: 2 in, 2 out]
            n149 = case shown="\"White Balance  **\"" w262 {
              tunnel: w261 -> [w268 w277 w286 w295 w304 _ w310]
              tunnel: w260 -> [w266 w274 w283 w292 w301 _ _]
              frame "Size  **" {
                n150 = Index Array(array=w266) -> (element=w265:cluster{string[]})  [unwired: 1 in]
                n151 = call <vilib>:"NT Read String.vi"("Name"=w268) -> ("String"=w267:string)  [unwired: 9 in, 1 out]
                n152 = Unbundle(w265) -> (w263:string[])
                n153 = Match First String(2:w263, 3:w267) -> (0:w264:i32)  [unwired: 1 out]
                n154 = property on="Test Ring" class="Ring (strict)"("Value"=w264, "Strings []"=w263) -> ()  [unwired: 2 in, 2 out]
                n155 = property on="Test Ring" class="Ring (strict)"("Visible"=TRUE) -> ()  [unwired: 2 in, 2 out]
                n156 = property on="Test Slider" class="Slide (strict)"("Visible"=FALSE) -> ()  [unwired: 2 in, 2 out]
              }
              frame "White Balance  **" {
                n157 = Index Array(array=w274, index=1) -> (element=w275:cluster{string[]})
                n158 = call <vilib>:"NT Read String.vi"("Name"=w277) -> ("String"=w276:string)  [unwired: 9 in, 1 out]
                n159 = Unbundle(w275) -> (w272:string[])
                n160 = Match First String(2:w272, 3:w276) -> (0:w271:i32)  [unwired: 1 out]
                n161 = property on="Test Ring" class="Ring (strict)"("Value"=w271, "Strings []"=w272) -> ()  [unwired: 2 in, 2 out]
                n162 = property on="Test Ring" class="Ring (strict)"("Visible"=TRUE) -> ()  [unwired: 2 in, 2 out]
                n163 = property on="Test Slider" class="Slide (strict)"("Visible"=FALSE) -> ()  [unwired: 2 in, 2 out]
              }
              frame "Exposure  **" {
                n164 = Index Array(array=w283, index=2) -> (element=w284:cluster{string[]})
                n165 = call <vilib>:"NT Read String.vi"("Name"=w286) -> ("String"=w285:string)  [unwired: 9 in, 1 out]
                n166 = Unbundle(w284) -> (w280:string[])
                n167 = Match First String(2:w280, 3:w285) -> (0:w281:i32)  [unwired: 1 out]
                n168 = property on="Test Ring" class="Ring (strict)"("Value"=w281, "Strings []"=w280) -> ()  [unwired: 2 in, 2 out]
                n169 = property on="Test Ring" class="Ring (strict)"("Visible"=TRUE) -> ()  [unwired: 2 in, 2 out]
                n170 = property on="Test Slider" class="Slide (strict)"("Visible"=FALSE) -> ()  [unwired: 2 in, 2 out]
              }
              frame "Exposure Priority  **" {
                n171 = Index Array(array=w292, index=3) -> (element=w293:cluster{string[]})
                n172 = call <vilib>:"NT Read String.vi"("Name"=w295) -> ("String"=w294:string)  [unwired: 9 in, 1 out]
                n173 = Unbundle(w293) -> (w289:string[])
                n174 = Match First String(2:w289, 3:w294) -> (0:w290:i32)  [unwired: 1 out]
                n175 = property on="Test Ring" class="Ring (strict)"("Value"=w290, "Strings []"=w289) -> ()  [unwired: 2 in, 2 out]
                n176 = property on="Test Ring" class="Ring (strict)"("Visible"=TRUE) -> ()  [unwired: 2 in, 2 out]
                n177 = property on="Test Slider" class="Slide (strict)"("Visible"=FALSE) -> ()  [unwired: 2 in, 2 out]
              }
              frame "Color Enable  **" {
                n178 = Index Array(array=w301, index=4) -> (element=w302:cluster{string[]})
                n179 = call <vilib>:"NT Read String.vi"("Name"=w304) -> ("String"=w303:string)  [unwired: 9 in, 1 out]
                n180 = Unbundle(w302) -> (w298:string[])
                n181 = Match First String(2:w298, 3:w303) -> (0:w299:i32)  [unwired: 1 out]
                n182 = property on="Test Ring" class="Ring (strict)"("Value"=w299, "Strings []"=w298) -> ()  [unwired: 2 in, 2 out]
                n183 = property on="Test Ring" class="Ring (strict)"("Visible"=TRUE) -> ()  [unwired: 2 in, 2 out]
                n184 = property on="Test Slider" class="Slide (strict)"("Visible"=FALSE) -> ()  [unwired: 2 in, 2 out]
              }
              frame Default {
                n185 = property on="Test Ring" class="Ring (strict)"("Visible"=FALSE) -> ()  [unwired: 2 in, 2 out]
                n186 = property on="Test Slider" class="Slide (strict)"("Visible"=FALSE) -> ()  [unwired: 2 in, 2 out]
              }
              frame "Brightness  **", "Color Level  **", "Compression  **", "FPS  **", "Sharpness  **" {
                n187 = call <vilib>:"NT Read Number.vi"("Name"=w310) -> ("Numeric"=w309:dbl)  [unwired: 9 in, 1 out]
                n188 = local write "Test Slider"(w309) -> ()
                n189 = property on="Test Slider" class="Slide (strict)"("Visible"=TRUE, "Scale.Maximum"=100.0 ("Scale.Range:Maximum")) -> ()  [unwired: 2 in, 2 out]
                n190 = property on="Test Ring" class="Ring (strict)"("Visible"=FALSE) -> ()  [unwired: 2 in, 2 out]
              }
            }
          }
        }
        n191 = property on="Progress" class="Clust (strict)"("Visible"=FALSE) -> ()  [unwired: 2 in, 2 out]
      }
      event "Test Name": Mouse Enter {
        # "Populate the ring with the list of tests"
        n192 = event-data() -> ()  [unwired: 1 in, 1 out]
        n193 = call <vilib>:"NT Read String Array.vi"("Name"="/TestMode/TestList") -> ("String Array"=w319:string[])  [unwired: 9 in, 1 out]
        n194 = Build Array (concatenate)("Select the test to run...", w319) -> (w318:string[])
        n195 = property on="Test Name" class="Ring (strict)"("Strings []"=w318) -> ()  [unwired: 2 in, 2 out]
      }
      event "Test Name": Value Change {
        w322 = FALSE ("Visible")
        # "Tell the robot the test name to run"
        n196 = event-data() -> ("NewVal"=w326:u16)  [unwired: 1 in]
        n197 = property on="Test Name" class="Ring (strict)"() -> ("Strings []"=w327:string[])  [unwired: 2 in, 2 out]
        n198 = local write "Progress"(T7 {"Test Progress"=0, "Test Progress Text"=""} ("Progress")) -> ()
        n199 = Index Array(array=w327, index=w326) -> (element=w325:string)
        n200 = call <vilib>:"NT Write String.vi"("String"=w325, "Name"="/TestMode/TestName") -> ()  [unwired: 9 in, 1 out]
        n201 = property on="Progress" class="Clust (strict)"("Visible"=TRUE) -> ()  [unwired: 2 in, 2 out]
        n202 = property on="Motor" class="Clust (strict)"("Visible"=w322) -> ()  [unwired: 2 in, 2 out]
        n203 = property on="Test Slider" class="Slide (strict)"("Visible"=w322) -> ()  [unwired: 2 in, 2 out]
        n204 = property on="On/Off" class="Bool (strict)"("Visible"=w322) -> ()  [unwired: 2 in, 2 out]
        n205 = property on="Rev/Fwd" class="Clust (strict)"("Visible"=w322) -> ()  [unwired: 2 in, 2 out]
        n206 = property on="Test Ring" class="Ring (strict)"("Visible"=w322) -> ()  [unwired: 2 in, 2 out]
      }
      event "Select Auto": Mouse Enter {
        # "Populate the combo box with the list of autonomous options"
        n207 = event-data() -> ()  [unwired: 1 in, 1 out]
        n208 = call <vilib>:"NT Read String Array.vi"("Name"="Auto List") -> ("String Array"=w329:string[])  [unwired: 9 in, 1 out]
        n209 = property on="Select Auto" class="CmbBox"("Strings[]"=w329) -> ()  [unwired: 2 in, 2 out]
      }
      event "Select Auto": Value Change {
        # "User modified the Auto Selection. Write to NT variable so robot knows."
        n210 = event-data() -> ("NewVal"=w333:string)  [unwired: 1 in]
        n211 = call <vilib>:"NT Write String.vi"("String"=w333, "Name"="Auto Selector") -> ()  [unwired: 9 in, 1 out]
      }
      event "Command Selection": Value Change {
        # "Get the params and show in table"
        n212 = event-data() -> ("NewVal"=w340:i32)  [unwired: 1 in]
        n213 = property on="Command Selection" class="MCListbox (strict)"() -> ("ItemNames"=w338:string[][])  [unwired: 2 in, 2 out]
        n214 = call <vilib>:"WPI_DashboardUpdate Command Params.vi"("NewVal"=w340, "Commands"=w338, "Param Tbl"=w339) -> ()  [unwired: 8 in, 1 out]
      }
      event "Execute Command": Value Change {
        # "Started one, Unique ID holds\nresponse"
        n215 = event-data() -> ()  [unwired: 1 in, 1 out]
        n216 = property on="Command Selection" class="MCListbox (strict)"() -> ("ItemNames"=w352:string[][])  [unwired: 2 in, 2 out]
        n217 = Index Array(array=w352, index (row)="Command Selection", index (col)=0) -> (element=w350:string)
        n218 = call <vilib>:"Invoke Commands.vi"("Command Params"="Command Params", "Function Name"=w350) -> ("Params"=w346:u8, "Started"=w345:bool)  [unwired: 7 in, 1 out]
        n219 = Array Subset(array="Command Params", length (row)=w346) -> (w347:string[][])  [unwired: 3 in]
        n220 = Select(t="Executing" ("Cmd Status"), s=w345, f="" ("Cmd Status")) -> (s? t:f=→"Cmd Status":string)
      }
      event "Command Selection": Double Click {
        n221 = event-data() -> ("Row"=w362:i32)  [unwired: 1 in]
        n222 = property on="Command Selection" class="MCListbox (strict)"() -> ("ItemNames"=w365:string[][])  [unwired: 2 in, 2 out]
        n223 = local read "Command Params"() -> (w360:string[][])
        n224 = Index Array(array=w365, index (row)=w362, index (col)=0) -> (element=w363:string)
        n225 = call <vilib>:"Invoke Commands.vi"("Command Params"=w360, "Function Name"=w363) -> ("Params"=w359:u8, "Started"=w354:bool)  [unwired: 7 in, 1 out]
        n226 = Array Subset(array=w360, length (row)=w359) -> (w358:string[][])  [unwired: 3 in]
        n227 = Select(t="Executing" ("Cmd Status"), s=w354, f="" ("Cmd Status")) -> (s? t:f=w355:string)
        n228 = local write "Cmd Status"(w355) -> ()
      }
      event "CheckList": Double Click {
        # "Shift clears all"
        # "Update symbols on the listbox"
        n229 = event-data() -> ("PlatMods.Shift"=w368:bool, "Row"=w370:i32)  [unwired: 1 in]
        n230 = case shown="True" w368 {
          tunnel: w370 -> [w374 _]
          tunnel: 1 -> [w373 _]
          frame False {
            n231 = property on="CheckList" class="LstBox (strict)"() -> ("Item Symbols"=w372:i32[])  [unwired: 2 in, 2 out]
            n232 = Replace Array Subset(array=w372, new element=w373, index=w374) -> (w371:i32[])
            n233 = property on="CheckList" class="LstBox (strict)"("Item Symbols"=w371) -> ()  [unwired: 2 in, 2 out]
          }
          frame True {
            w375 = 0 ("Top Row")
            n234 = property on="CheckList" class="LstBox (strict)"() -> ("Number of Rows"=w377:u32)  [unwired: 2 in, 2 out]
            n235 = Initialize Array(0, w377) -> (w376:i32[])
            n236 = property on="CheckList" class="LstBox (strict)"("Top Row"=w375, "Value"=w375, "Item Symbols"=w376) -> ()  [unwired: 2 in, 2 out]
          }
        }
      }
      event "CheckList": Key Down {
        # "Update symbols on the listbox\nLeft and right keys check and uncheck"
        n237 = event-data() -> ("VKey"=w382:T22)  [unwired: 1 in]
        n238 = case shown="\"Left\", \"Right\"" w382 {
          selector: w382 -> [w387 _]
          tunnel: eventvkey."Left" ("VKey") -> [w385 _]
          frame "Left", "Right" {
            n239 = Equal?(x=w385, y=w387) -> (x = y?=w386:bool)
            n240 = Select(t=0, s=w386, f=1) -> (s? t:f=w388:i32)
            n241 = property on="CheckList" class="LstBox (strict)"() -> ("Item Symbols"=w391:i32[])  [unwired: 2 in, 2 out]
            n242 = Replace Array Subset(array=w391, new element=w388, index="CheckList") -> (w390:i32[])
            n243 = property on="CheckList" class="LstBox (strict)"("Item Symbols"=w390) -> ()  [unwired: 2 in, 2 out]
          }
          frame Default {
          }
        }
      }
      event "DB Camera Config": Value Change {
        # "Show or hide the cluster of controls, store in ini file"
        n244 = event-data() -> ("NewVal"=w396:bool)  [unwired: 1 in]
        n245 = case shown="False" w396 {
          tunnel: w395 -> [w405 _]
          tunnel: [w398 w416] -> w394
          tunnel: w393 -> [w397 w416]
          frame False {
            w412 = "Camera"
            w415 = FALSE ("Visible")
            n246 = local read "Camera Settings"() -> (w404:T2)
            n247 = Index Array(array=w405) -> (element=w408:cluster{string[]})  [unwired: 1 in]
            n248 = Unbundle(w404) -> ("Frame Rate"=w403:i32, "Compression"=w402:i32, "Size"=w406:u16)
            n249 = Unbundle(w408) -> (w407:string[])
            n250 = Index Array(array=w407, index=w406) -> (element=w401:string)
            n251 = call-poly <vilib>:"Write Key.vi"("section"=w412, "value"=w401, "key"="Size", "refnum"=w397) -> ("refnum out"=w414:T20)  [unwired: 2 in, 5 out]
            n252 = call-poly <vilib>:"Write Key.vi"("section"=w412, "value"=w403, "key"="FrameRate", "refnum"=w414) -> ("refnum out"=w413:T20)  [unwired: 1 in, 6 out]
            n253 = property on="Camera Settings" class="Clust (strict)"("Visible"=w415) -> ()  [unwired: 2 in, 2 out]
            n254 = local write "DB Camera Config"(w415) -> ()
            n255 = call-poly <vilib>:"Write Key.vi"("section"=w412, "value"=w402, "key"="Compression", "refnum"=w413) -> ("refnum out"=w399:T20)  [unwired: 1 in, 6 out]
            n256 = call <vilib>:"Close Config Data.vi"("refnum"=w399) -> ("file path"=w400:path)  [unwired: 2 in, 8 out]
            n257 = call <vilib>:"Open Config Data.vi"("configuration file path"=w400) -> ("refnum"=w398:T20)  [unwired: 8 in, 2 out]
          }
          frame True {
            n258 = property on="Camera Settings" class="Clust (strict)"("Visible"=TRUE) -> ()  [unwired: 2 in, 2 out]
          }
        }
      }
      event "Camera Settings": Value Change {
        # "Update summary string when any elements of DB camera change"
        n259 = event-data() -> ("NewVal"=w430:T2)  [unwired: 1 in]
        n260 = Index Array(array=w426) -> (element=w425:cluster{string[]})  [unwired: 1 in]
        n261 = Unbundle(w430) -> ("Frame Rate"=w421:i32, "Compression"=w420:i32, "Size"=w423:u16)
        n262 = Unbundle(w425) -> (w424:string[])
        n263 = Index Array(array=w424, index=w423) -> (element=w422:string)
        n264 = Format Into String(format string="%s   %dfps   %d%%", w422, w421, w420) -> (resulting string=w427:string)  [unwired: 2 in, 1 out]
        n265 = Build Array(w427) -> (w428:string[])
        n266 = property on="DB Camera Config" class="Bool (strict)"("Strings [4]"=w428) -> ()  [unwired: 2 in, 2 out]
      }
      event "Motor.Enable": Value Change {
        # "When the test mode otor enable helper is set, update that\ntree row item's value"
        n267 = event-data() -> ("NewVal"=w437:bool)  [unwired: 1 in]
        n268 = Unbundle("Motor") -> ("Value"=w436:dbl)  [unwired: 1 out]
        n269 = Select(t=w436, s=w437, f=0.0) -> (s? t:f=w434:dbl)
        n270 = call <vilib>:"NT Write Number.vi"("Numeric"=w434, "Name"=w433) -> ()  [unwired: 9 in, 1 out]
      }
      event "Test Slider": Value Change {
        # "When the test mode slider helper is set, update that\ntree row item's value"
        n271 = event-data() -> ("NewVal"=w441:dbl)  [unwired: 1 in]
        n272 = call <vilib>:"NT Write Number.vi"("Numeric"=w441, "Name"=w442) -> ()  [unwired: 9 in, 1 out]
      }
      event "On/Off": Value Change {
        # "When the test mode on/off helper value is set, update that\ntree row item's value"
        n273 = event-data() -> ("NewVal"=w447:bool)  [unwired: 1 in]
        n274 = Boolean To (0,1)(Boolean=w447) -> (0, 1=w446:i16)
        n275 = call <vilib>:"NT Write Number.vi"("Numeric"=w446, "Name"=w445) -> ()  [unwired: 9 in, 1 out]
      }
      event "Rev/Fwd": Value Change {
        # "When the test mode helper value for relays is set, update that\ntree row item's value"
        n276 = event-data() -> ("NewVal.Forward"=w456:bool, "NewVal.Reverse"=w455:bool)  [unwired: 1 in]
        n277 = Boolean To (0,1)(Boolean=w456) -> (0, 1=w452:i16)
        n278 = Boolean To (0,1)(Boolean=w455) -> (0, 1=w454:i16)
        n279 = Negate(x=w454) -> (-x=w453:i16)
        n280 = Add(x=w452, y=w453) -> (x+y=w451:i16)
        n281 = call <vilib>:"NT Write Number.vi"("Numeric"=w451, "Name"=w450) -> ()  [unwired: 9 in, 1 out]
      }
      event "Test Ring": Value Change {
        # "When a test mode helper value is selected from the ring,\nset the tree item's variable to the string value"
        n282 = event-data() -> ("NewVal"=w461:u16)  [unwired: 1 in]
        n283 = property on="Test Ring" class="Ring (strict)"() -> ("Strings []"=w462:string[])  [unwired: 2 in, 2 out]
        n284 = Index Array(array=w462, index=w461) -> (element=w460:string)
        n285 = call <vilib>:"NT Write String.vi"("String"=w460, "Name"=w459) -> ()  [unwired: 9 in, 1 out]
      }
      event "Rec Mode": Value Change {
        # "Update globals for recording mode and path to read log from.\nClear when logging and let NetworkTables set path for vision to\nuse."
        n286 = event-data() -> ("NewVal"=w474:enum32{"Stop", "Record", "Playback"})  [unwired: 1 in]
        n287 = global write "WPI_DashboardLogging Global.vi" "Logging Filename"(path "") -> ()
        n288 = global write "WPI_DashboardLogging Global.vi" "Recording"(w474) -> ()
        n289 = case shown="\"Playback\"" w474 {
          tunnel: w473 -> [_ w476 w485]
          tunnel: [_ _ w484] -> w470
          tunnel: [_ _ w483] -> _
          tunnel: w468 -> [_ _ w481]
          tunnel: cluster{i32, i32} {-250, 170} -> [_ _ w480]
          tunnel: [_ _ T23 {"Image Size"=TRUE, "Image Type"=TRUE, "Pixel Value"=TRUE, "ROI Information"=TRUE, "Zoom Factor"=FALSE} ("Image Information Shown:All Elements")] -> w466
          tunnel: [_ _ TRUE ("Zoom Factor")] -> w465
          tunnel: w464 -> [_ _ w477]
          frame Default {
          }
          frame "Stop", "Record" {
            # "Place Window too"
            n290 = invoke class="VI" method="FP.Close"(reference=w476) -> (reference out=w475:refnum<vi>)  [unwired: 2 in, 2 out]
            n291 = invoke class="VI" method="Abort VI"(reference=w475) -> ()  [unwired: 2 in, 3 out]
          }
          frame "Playback" {
            n292 = call "Open Playback Panel.vi"("Offset"=w480, "DB VI Ref"=w481, "Playback in"=w485) -> ("Playback out"=w482:refnum<vi>)  [unwired: 8 in]
            n293 = register-events(w482, w477) -> (reference out=w484:refnum<event-registration>, error out=w483:errorcluster)  [unwired: 2 in]
          }
        }
        n294 = property on="Camera Image" class="ImageControl"("Image Information Shown"=w466, "Image Information Visible"=w465) -> ()  [unwired: 2 in, 2 out]
        n295 = call <vilib>:"WPI_DashboardNT Log FieldName Cache.vi"("Operation"=enum16{"Lookup/Add", "Index", "Clear"}."Clear") -> ()  [unwired: 8 in, 3 out]
      }
      event Panel Close {
        w487 = enum32{"Stop", "Record", "Playback"}."Stop" ("Rec Mode")
        # "Playback window has been closed, abort"
        n296 = event-data() -> ()  [unwired: 1 in, 4 out]
        n297 = local write "Rec Mode"(w487) -> ()
        n298 = global write "WPI_DashboardLogging Global.vi" "Recording"(w487) -> ()
      }
      event Panel Close {
        # "Abort playback window and ourself"
        n299 = event-data() -> ()  [unwired: 1 in, 4 out]
        n300 = invoke class="VI" method="FP.Close"(reference=w493) -> (reference out=w492:refnum<vi>)  [unwired: 2 in, 2 out]
        n301 = invoke class="VI" method="Abort VI"(reference=w492) -> (error out=w491:errorcluster)  [unwired: 2 in, 2 out]
        n302 = invoke class="VI" method="Abort VI"(error in=w491) -> ()  [unwired: 2 in, 3 out]
      }
      event User Event {
        n303 = event-data() -> ("IDs"=w501:cluster{"RPC field ID":u16, "Unique ID":u16}, "String"=w500:string)  [unwired: 1 in]
        n304 = Bundle("IDs"=w501, "String"=w500) -> (w499:T9)  [unwired: 1 in]
        n305 = call <vilib>:"Retrieve RPC Response.vi"("RPC Response"=w499) -> ("Output"=w496:string[][])  [unwired: 10 in]
        n306 = Build Array (concatenate)(w494, w496) -> (w495:string[][])
        n307 = local write "Command Params"(w495) -> ()
        n308 = local write "Cmd Status"("" ("Cmd Status")) -> ()
      }
      event "Vision": Value Change {
        # "Enable/Disable Compression slider.\nHW USB is hard-coded into the camera"
        n309 = event-data() -> ("NewVal"=w508:u16)  [unwired: 1 in]
        n310 = Equal?(x=w508, y=u32 2 ("milliseconds to wait")) -> (x = y?=w506:bool)
        n311 = Select(t=T24."Disabled and Grayed Out" ("Disabled"), s=w506, f=T24."Enabled" ("Disabled")) -> (s? t:f=w503:T24)
        n312 = property on="Compression" class="Slide (strict)"("DisabledEnum"=w503) -> ()  [unwired: 2 in, 2 out]
      }
      event "Tree": Double Click {
        n313 = event-data() -> ("PlatMods"=w513:T27, "Tag"=w512:string)  [unwired: 1 in]
        n314 = Unbundle(w513) -> ("Shift"=w511:bool)  [unwired: 4 out]
        n315 = Not(x=w511) -> (.not. x?=w510:bool)
        n316 = call <vilib>:"NT Update Persistence.vi"("Persistence"=w510, "Name"=w512) -> ()  [unwired: 9 in, 1 out]
      }
    }
  }
  n317 = while {
    tunnel: w52 -> [w517]
    i -> [w520]
    stop <- FALSE stop-if-true
    n318 = Wait (ms)(milliseconds to wait=u32 100) -> ()  [unwired: 1 out]
    n319 = case shown="\"Playback\"" "Rec Mode" {
      tunnel: w520 -> [_ _ w535]
      tunnel: [u32 2829099 ("Base Color") u32 11141120 ("Target Color") w524] -> w516
      frame "Stop", Default {
        # "Reset the color, extra updates don't cost much"
      }
      frame "Record" {
      }
      frame "Playback" {
        # "Playback"
        n320 = Quotient & Remainder(x=w535, y=u32 50 ("milliseconds to wait")) -> (x-y*floor(x/y)=w531:u32)  [unwired: 1 out]
        n321 = Divide(x=w531, y=u32 50 ("milliseconds to wait")) -> (x/y=w528:dbl)
        n322 = Multiply(x=6.283185307179586, y=w528) -> (x*y=w533:dbl)
        n323 = Sine(x=w533) -> (sin(x)=w532:dbl)
        n324 = Absolute Value(x=w532) -> (abs(x)=w525:dbl)
        n325 = call "Interpolate RGB Color.vi"("Proportion"=w525, "Target Color"=u32 30976, "Base Color"=u32 2829099) -> ("Result Color"=w524:u32)  [unwired: 8 in]
      }
    }
    n326 = property class="Pane"(reference=w517, "PaneColor"=w516) -> ()  [unwired: 1 in, 2 out]
  }
  n327 = local write "Dashboard Tab"(T1."Drive" ("Dashboard Tab")) -> ()
  n328 = call "Build XY Graph"("Enable"="Enable_Camera", "Reset"="Reset_Camera", "Y Input"="Position_y", "X Input"="Position_x") -> ("XY Graph"=→"XY Graph":cluster{"X":dbl[], "Y":dbl[]}[])  [unwired: 6 in, 1 out]
  n329 = property on="On/Off" class="Bool (strict)"("Visible"=w20) -> ()  [unwired: 2 in, 2 out]
  n330 = property on="Motor" class="Clust (strict)"("Visible"=w20) -> ()  [unwired: 2 in, 2 out]
  n331 = property on="Progress" class="Clust (strict)"("Visible"=w20) -> ()  [unwired: 2 in, 2 out]
  n332 = property on="Test Ring" class="Ring (strict)"("Visible"=w20) -> ()  [unwired: 2 in, 2 out]
  n333 = property on="Rev/Fwd" class="Clust (strict)"("Visible"=w20) -> ()  [unwired: 2 in, 2 out]
  n334 = property on="Camera Settings" class="Clust (strict)"("Visible"=w20) -> ()  [unwired: 2 in, 2 out]
  n335 = while {
    tunnel: u16 1741 ("timeout ms (25000)") -> [w537]
    stop <- FALSE stop-if-true
    n336 = TCP Create Listener(10:w537) -> (0:w536:errorcluster, 3:w538:refnum<k5>)  [unwired: 4 in, 1 out]
    n337 = case shown="No Error" w536 {
      selector: w536 -> [w540 _]
      tunnel: w538 -> [w541 _]
      frame No Error {
        n338 = while {
          tunnel: w541 -> [w544]
          tunnel: w540 -> [w543]
          stop <- FALSE stop-if-true
          n339 = TCP Wait On Listener(8:w543, 11:w544) -> (0:w545:errorcluster, 4:w546:refnum<k5>)  [unwired: 2 in, 3 out]
          n340 = local write "TCP"(w546) -> ()
          n341 = case shown="No Error" w545 {
            frame No Error {
            }
            frame Error {
              n342 = Wait (ms)(milliseconds to wait=u32 1000) -> ()  [unwired: 1 out]
            }
          }
        }
      }
      frame Error {
        n343 = Wait (ms)(milliseconds to wait=u32 1000) -> ()  [unwired: 1 out]
      }
    }
  }
  n344 = local write "DB Camera Config"(w20) -> ()
  n345 = local write "Command Params"(string[][] [] ("Command Params")) -> ()
  n346 = global write "WPI_DashboardLogging Global.vi" "Recording"(w46) -> ()
  n347 = local write "Command Selection"(u16 0 ("milliseconds to wait")) -> ()
  n348 = local write "Rec Mode"(w46) -> ()
